vi "SubPanel_DataCollection_Rev11_v3.vi"(0 "DCPowerInformationClusterArray_Input":T1(array[cluster]), 1 "VISAPowerInfoInputArray":T7(array[cluster]), 2 "Run Data SubPanel Input":T6, 3 "RF Block Parameters":T5, 4 "Oscilloscope Info Array":T4(array[cluster]) {"vertical coupling" items=["AC", "DC", "Ground"]}, 6 "New Run?":bool, 7 "error in":errorcluster) -> (20 "DCPowerInformationClusterArray_Output":T1(array[cluster]), 21 "VISAPowerInfoInputOutput":T7(array[cluster]), 22 "Run Data SubPanel Output":T6, 23 "RF Block Parameters Output":T5, 24 "Oscilloscope Info Array Output":T4(array[cluster]) {"vertical coupling" items=["AC", "DC", "Ground"]}, 25 "Reinitialize?":bool, 26 "Data Was Collected?":bool, 27 "error out":errorcluster)   [LabVIEW 2019]
uses:
  Controls/QueueDataControl.ctl
  Controls/DataBlockControl.ctl
  Controls/QueueDataControl_V2.ctl
  Controls/RFBlockControl.ctl
  <instrlib>/niScope/Controls/niScope vertical coupling.ctl
panel:
  out "DCPowerInformationClusterArray_Input 2":T1(array[cluster])
  out "Forced Exit":bool
  out "output cluster":T2
  out "Full Run Information":string
  out "Ready For Next Run?":bool
  in  "Next Run":bool
  out "Latchup Output Data":dbl[][](array[numeric])
  out "Recording Data":bool
  out "Current 2":waveform(dbl)[](graph)
  out "Voltage 2":waveform(dbl)[](graph)
  out "Current":waveform(dbl)[](graph)
  out "Voltage":waveform(dbl)[](graph)
  in  "End Collecting":bool
  in  "Record Data Toggle":bool
  out "error of collection":errorcluster
  in  "force exit SubVI":bool
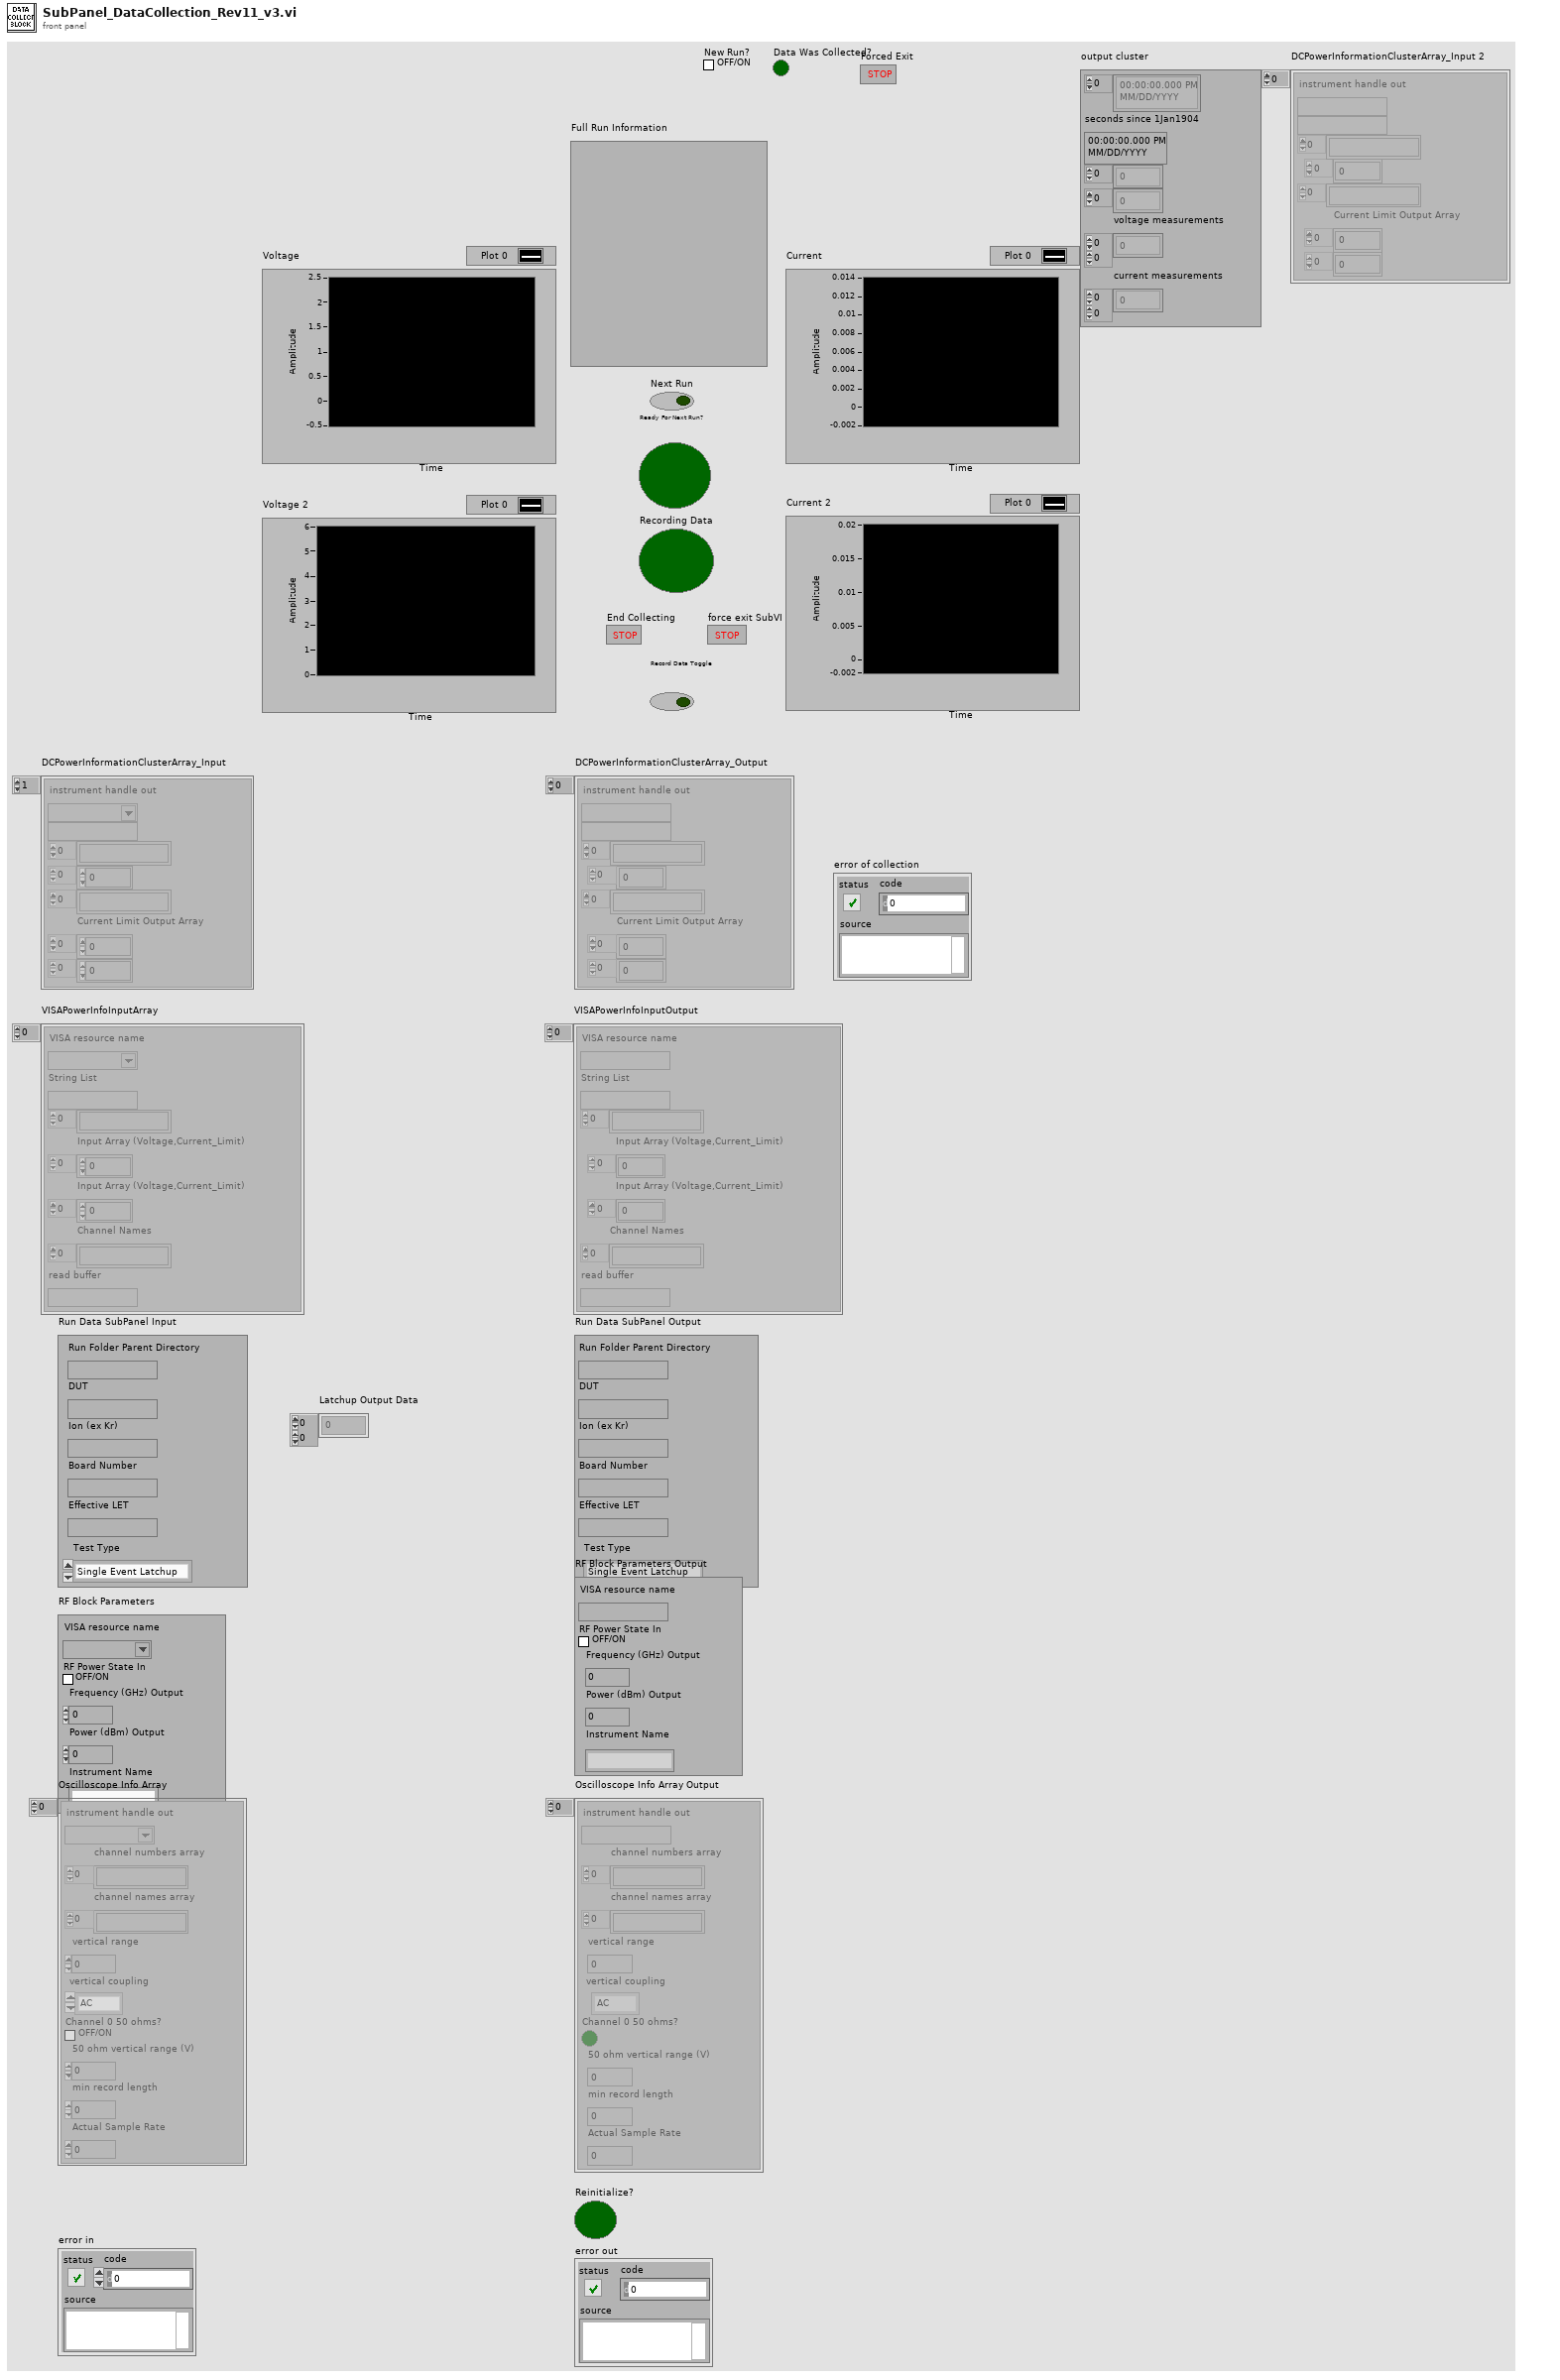
[diagram p1: front panel]
types:
  T1 = cluster{"instrument handle out":refnum<k15>, string, string[], dbl[], string[], "Current Limit Output Array":dbl[], dbl[]}[]
  T2 = cluster{timestamp[], "seconds since 1Jan1904":timestamp, dbl[], i32[], "voltage measurements":dbl[][], "current measurements":dbl[][]}
  T3 = typedef "niScope vertical coupling.ctl" = i32
  T4 = cluster{"instrument handle out":refnum<k15>, "channel numbers array":string[], "channel names array":string[], "vertical range":dbl, "vertical coupling":T3, "Channel 0 50 ohms?":bool, "50 ohm vertical range (V)":dbl, "min record length":i32, "Actual Sample Rate":dbl}[]
  T5 = typedef "RFBlockControl.ctl" = cluster{"VISA resource name":refnum<visa-resource-name>, "RF Power State In":bool, "Frequency (GHz) Output":dbl, "Power (dBm) Output":dbl, "Instrument Name":string}
  T6 = typedef "DataBlockControl.ctl" = cluster{"Run Folder Parent Directory":path, "DUT":string, "Ion (ex Kr)":string, "Board Number":string, "Effective LET":string, "Test Type":enum16{"Single Event Latchup", "Single Event Transient", "Single Event Upset"}}
  T7 = cluster{"VISA resource name":refnum<visa-resource-name>, "String List":string, string[], "Input Array (Voltage,Current_Limit)":dbl[], "Input Array (Voltage,Current_Limit)":dbl[], "Channel Names":string[], "read buffer":string}[]
  T8 = typedef "QueueDataControl_V2.ctl" = cluster{"Time Stamp Array":timestamp[], "Initial Time":timestamp, "dt measurement array":dbl[], "samples per capture":i32[], "voltage measurements":dbl[][], "current measurements":dbl[][]}
  T9 = cluster{"IVI Refnum out":refnum<k15>, string, "voltage level channel 23":dbl, "Channel Name 23":string, "Current Limit":dbl, "Measure Record dt":dbl, string}[]
  T10 = typedef "QueueDataControl.ctl" = cluster{"Rolling Timer":timestamp, "Initial Time":timestamp, "dt between samples":dbl[], "number of samples per fetch":i32[], "voltage measurements":dbl[][], "current measurements":dbl[][]}
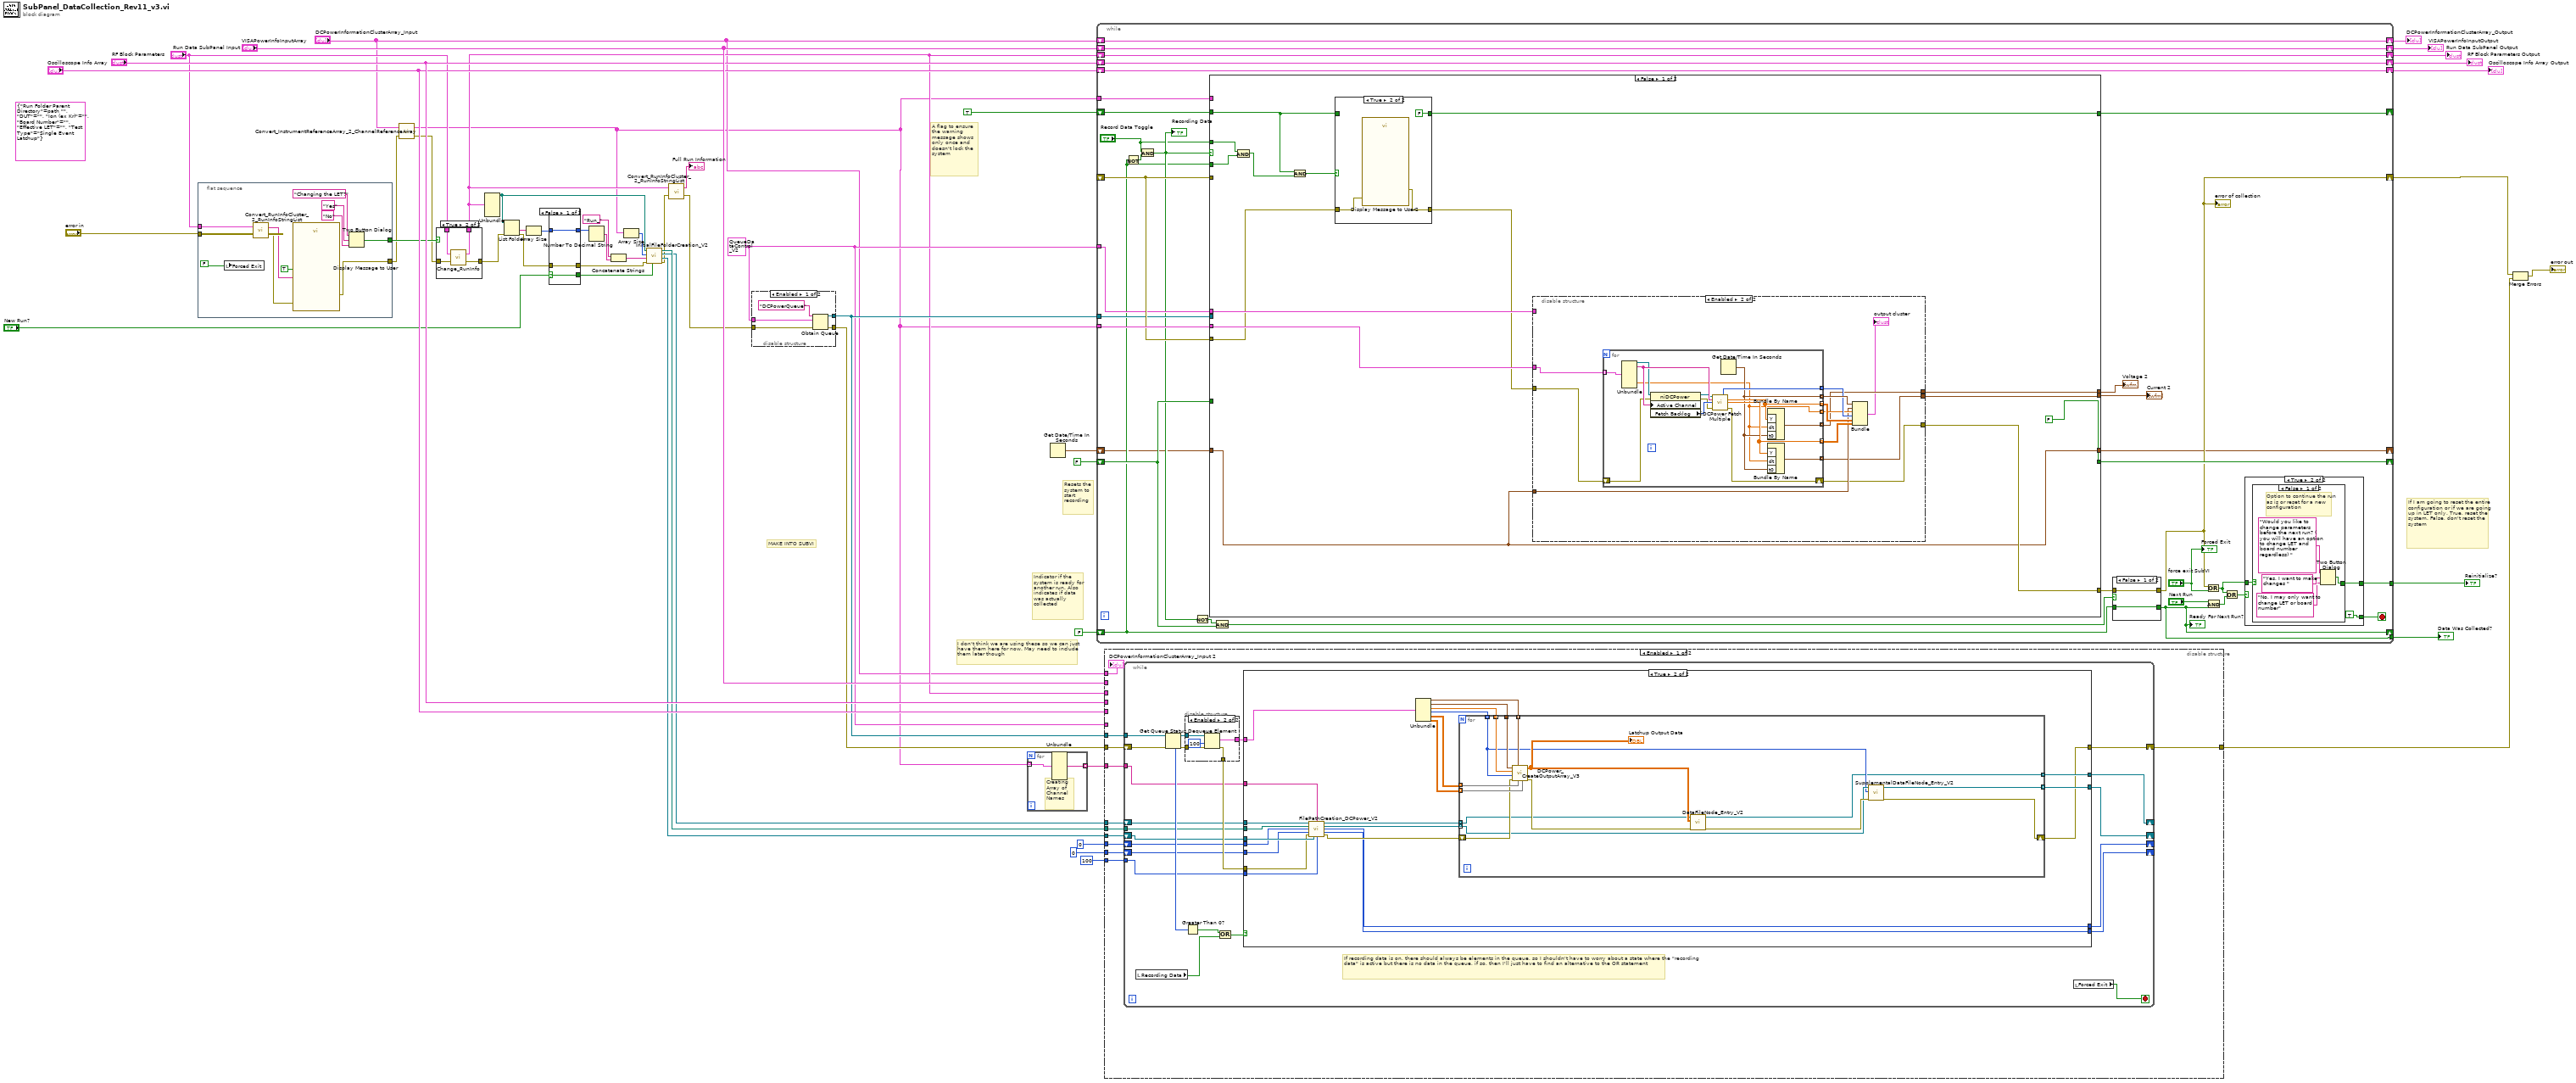
[diagram p0: block diagram]
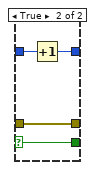
[diagram p2: hidden frame]
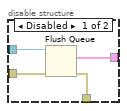
[diagram p5: hidden frame]
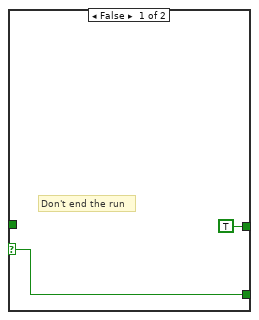
[diagram p8: hidden frame]
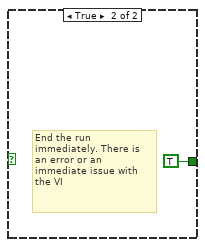
[diagram p9: hidden frame]
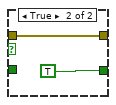
[diagram p10: hidden frame]
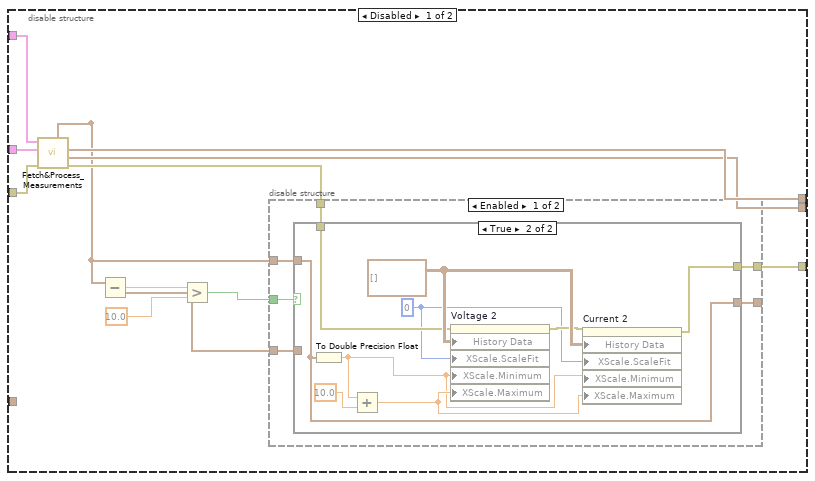
[diagram p11: hidden frame]
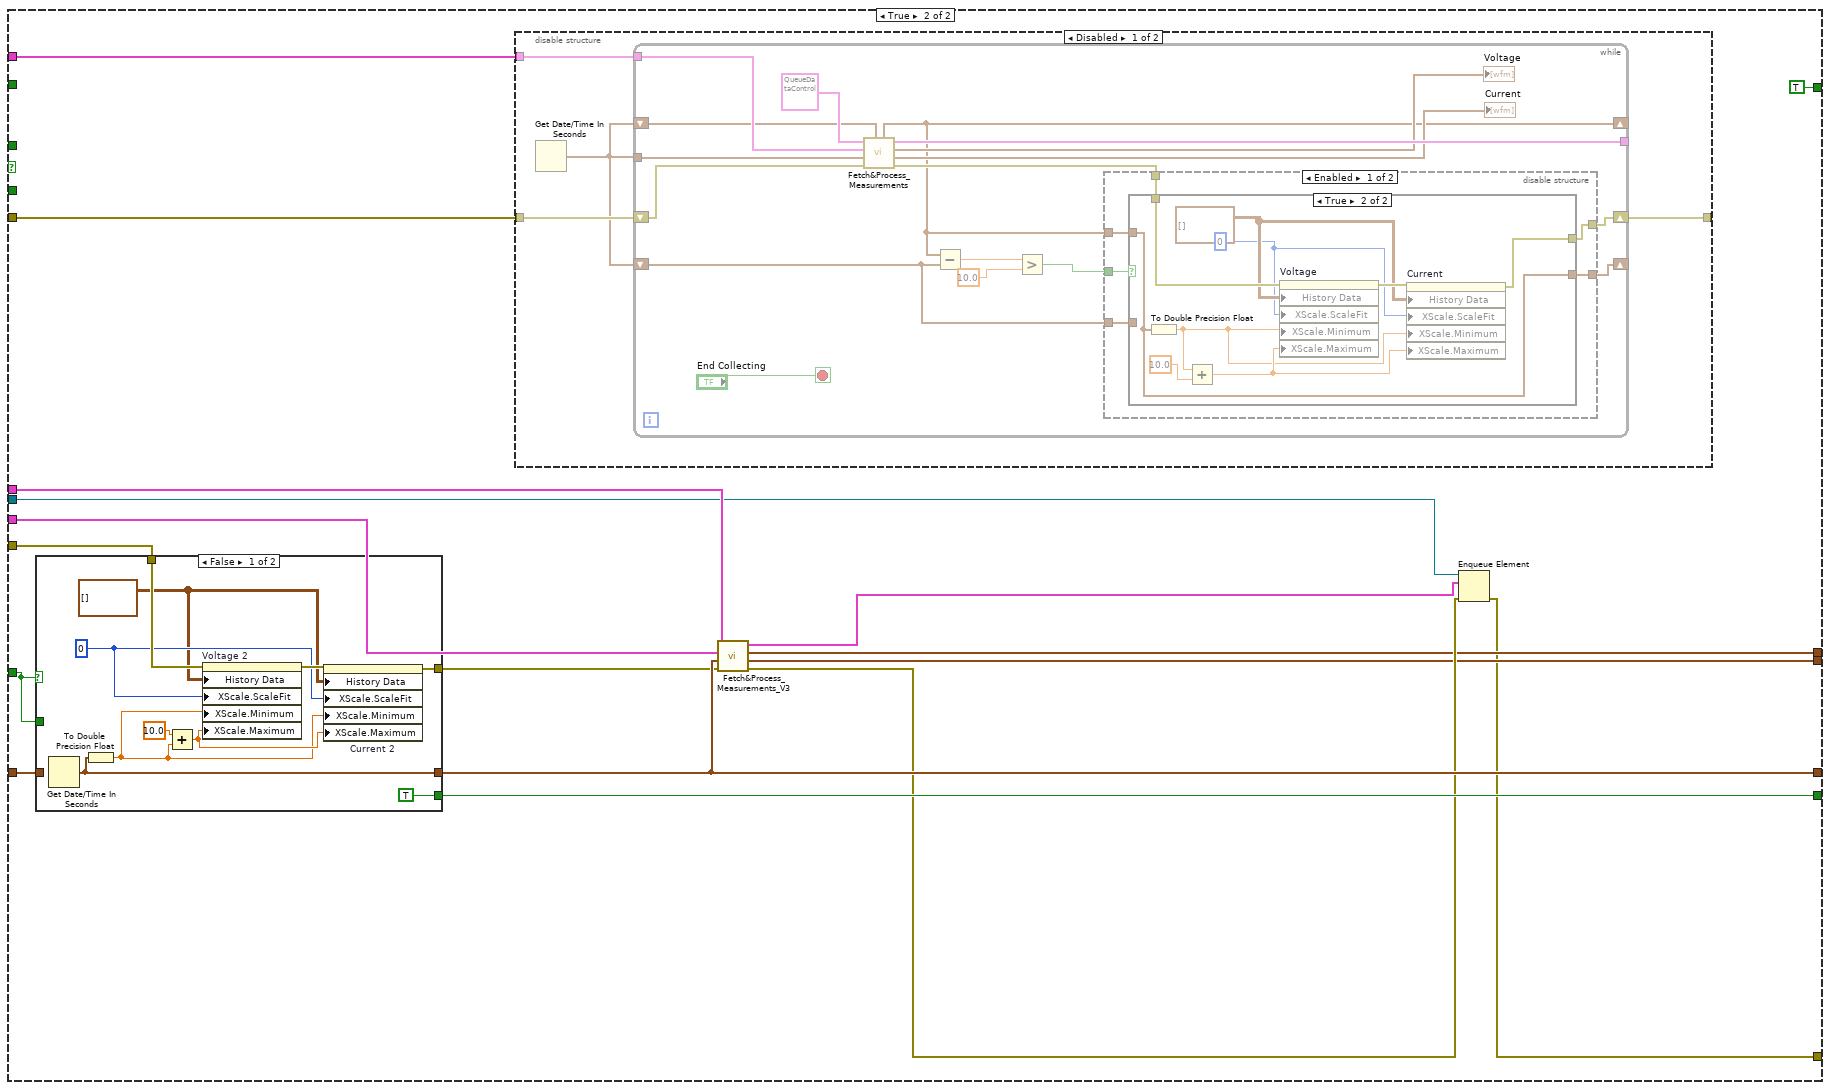
[diagram p15: hidden frame]
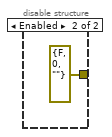
[diagram p19: hidden frame]
diagram:
  w32 = T8 {"Time Stamp Array"=[], "Initial Time"=timestamp(0 s since 1904-01-01), "dt measurement array"=[], "samples per capture"=[], "voltage measurements"=[], "current measurements"=[]} ("DCPowerDataQueueControl_V2")
  (unwired) T6 {"Run Folder Parent Directory"=path "", "DUT"="", "Ion (ex Kr)"="", "Board Number"="", "Effective LET"="", "Test Type"=enum."Single Event Latchup"} ("Run Data Configuration")
  # "I don't think we are using these so we can just have them here for now. May need to include them later though"
  # "Indicator if the system is ready for another run. Also indicates if data was actually collected"
  # "Resets the system to start recording"
  # "A flag to ensure the warning message shows only once and doesn't lock the system"
  # "If I am going to reset the entire configuration or if we are going up in LET only. True, reset the system. False, don't reset the system"
  # "MAKE INTO SUBVI"
  n1 = flat-sequence {
    tunnel: [w58] -> w26
    tunnel: "error in" -> [w57]
    tunnel: [w62] -> w36
    tunnel: "Run Data SubPanel Input" -> [w55]
    frame #0 {
      n2 = local write "Forced Exit"(FALSE ("Forced Exit")) -> ()
      n3 = call "Convert_RunInfoCluster_2_RunInfoStringList.vi"("error in"=w57, "Run Data SubPanel Input"=w55) -> ("error output"=w56:errorcluster, "Run Data Output"=w54:string)
      n4 = call "Display Message to User"("error in (no error)"=w56, "Enable"=TRUE, "Message"=w54) -> ("error out"=w58:errorcluster)  [unwired: 7 in, 1 out]
      n5 = Two Button Dialog(message="Changing the LET?", 1:"No" ("F button name (\"Cancel\")"), 2:"Yes" ("T button name (\"OK\")")) -> (T button?=w62:bool)
    }
  }
  n6 = call "Convert_InstrumentReferenceArray_2_ChannelReferenceArray.vi"("error in (no error)"=w26, "DCPowerInformationClusterArray_Input"="DCPowerInformationClusterArray_Input") -> ("error out"=w24:errorcluster, "DCPowerInformation_byChannel"=w7:T9)
  n7 = case shown="True" w36 {
    tunnel: "Run Data SubPanel Input" -> [w64 w68]
    tunnel: [w64 w67] -> w31
    tunnel: [w63 w66] -> w28
    tunnel: w24 -> [w63 w65]
    frame False {
    }
    frame True {
      n8 = call "Change_RunInfo.vi"("error in (no error)"=w65, "Run Data SubPanel in"=w68) -> ("error out"=w66:errorcluster, "Run Data SubPanel out"=w67:T6)
    }
  }
  n9 = Unbundle(w31) -> ("Run Folder Parent Directory"=w29:path)  [unwired: 5 out]
  n10 = List Folder(path=w29, error in=w28) -> (folder names=w30:string[], error out=w8:errorcluster)  [unwired: 2 in, 2 out]
  n11 = Array Size(array=w30) -> (size(s)=w11:i32)
  n12 = case shown="False" "New Run?" {
    selector: "New Run?" -> [w70 w73]
    tunnel: [w71 w75] -> w12
    tunnel: w11 -> [w71 w74]
    tunnel: [w70 w73] -> w10
    tunnel: [w69 w72] -> w9
    tunnel: w8 -> [w69 w72]
    frame False {
    }
    frame True {
      n13 = Increment(x=w74) -> (x+1=w75:i32)
    }
  }
  n14 = Number To Decimal String(number=w12) -> (decimal integer string=w16:string)  [unwired: 1 in]
  n15 = Concatenate Strings("Run_", w16) -> (w27:string)
  n16 = Array Size(array=w7) -> (size(s)=w6:i32)
  n17 = call "InitialFileFolderCreation_V2.vi"("New Run?"=w10, "error in (no error)"=w9, "Run Number"=w27, "DCPowerArrayClusterSize"=w6, "base path"=w29) -> ("error out"=w5:errorcluster, "SupplementalDataFileReferenceObjectArray"=w20:refnum<file>[], "DataFileReferenceObjectArray"=w21:refnum<file>[], "created path"=w22:path)  [unwired: 3 in]
  n18 = call "Convert_RunInfoCluster_2_RunInfoStringList.vi"("error in"=w5, "Run Data SubPanel Input"=w31) -> ("error output"=w4:errorcluster, "Run Data Output"=→"Full Run Information":string)
  n19 = disable-structure shown="Enabled" {
    disable-tunnel: w4 -> [w79 w81]
    disable-tunnel: [w78 w81] -> w41
    disable-tunnel: w32 -> [w77 _]
    disable-tunnel: [w76 _] -> w42
    frame Enabled {
      n20 = Obtain Queue(name (unnamed)="DCPowerQueue", element data type=w77, error in (no error)=w79) -> (queue out=w76:refnum<queue>, error out=w78:errorcluster)  [unwired: 2 in, 1 out]
    }
    frame Disabled {
    }
  }
  n21 = for {
    tunnel: w7 -> [w83] mode=indexing
    tunnel: [w82] -> w23 mode=indexing
    # "Creating Array of Channel Names"
    n22 = Unbundle(w83) -> ("Channel Name 23"=w82:string)  [unwired: 6 out]
  }
  n23 = Get Date/Time In Seconds() -> (seconds since 1Jan1904=w33:timestamp)
  n24 = while {
    shift-right: [w113] -> w51
    shift-left: "DCPowerInformationClusterArray_Input" -> [w113]
    shift-right: [w117] -> w50
    shift-left: "VISAPowerInfoInputArray" -> [w117]
    shift-right: [w116] -> w49
    shift-left: w31 -> [w116]
    shift-right: [w115] -> w48
    shift-left: "RF Block Parameters" -> [w115]
    shift-right: [w114] -> w47
    shift-left: "Oscilloscope Info Array" -> [w114]
    shift-right: [w96] -> w2
    shift-left: _ -> [w110]
    tunnel: w7 -> [w112]
    tunnel: w7 -> [w111]
    shift-right: [w107] -> _
    shift-left: FALSE -> [w103]
    tunnel: w32 -> [w106]
    tunnel: w42 -> [w105]
    shift-right: [w84] -> _
    shift-left: FALSE -> [w89]
    tunnel: [w93] -> w40
    shift-right: [w87] -> _
    shift-left: TRUE ("x .and. y?") -> [w88]
    shift-right: [w85] -> _
    shift-left: w33 -> [w86]
    tunnel: [w84] -> w14
    stop <- w94 stop-if-true
    n25 = Not(x=w89) -> (.not. x?=w91:bool)
    n26 = And(x="Record Data Toggle", y=w91) -> (x .and. y?=w92:bool)
    "Recording Data" <- w92
    n27 = Not(x=w92) -> (.not. x?=w104:bool)
    n28 = case shown="False" w92 {
      tunnel: w110 -> [_ w228]
      tunnel: w112 -> [_ w227]
      tunnel: w111 -> [w146 w225]
      tunnel: w110 -> [w140 w222]
      tunnel: [w143 w213] -> w109
      tunnel: [w144 w214] -> w108
      tunnel: w106 -> [w145 w218]
      tunnel: w103 -> [_ w219]
      tunnel: [FALSE w220] -> w107
      tunnel: w105 -> [_ w217]
      tunnel: [w141 w212] -> w101
      tunnel: "Record Data Toggle" -> [w137 _]
      tunnel: w89 -> [w138 _]
      tunnel: w88 -> [w133 _]
      tunnel: [w134 TRUE] -> w87
      tunnel: w86 -> [w132 w224]
      tunnel: [w132 w223] -> w85
      frame False {
        n29 = And(x=w137, y=w138) -> (x .and. y?=w136:bool)
        n30 = And(x=w133, y=w136) -> (x .and. y?=w135:bool)
        n31 = case shown="True" w135 {
          tunnel: [w208 w210] -> w139
          tunnel: w140 -> [w208 w211]
          tunnel: [w207 FALSE] -> w134
          tunnel: w133 -> [w207 _]
          frame False {
          }
          frame True {
            n32 = call "Display Message to User2"("error in (no error)"=w211) -> ("error out"=w210:errorcluster)  [unwired: 9 in, 1 out]
          }
        }
        n33 = disable-structure shown="Enabled" {
          disable-tunnel: w146 -> [w156 w186]
          disable-tunnel: w145 -> [w155 _]
          disable-tunnel: [w151 w184] -> w144
          disable-tunnel: [w150 w183] -> w143
          disable-tunnel: [w148 w182] -> w141
          disable-tunnel: w139 -> [w147 w181]
          disable-tunnel: w132 -> [_ w185]
          frame Disabled {
            n34 = call "Fetch&Process_Measurements.vi"("error in (no error)"=w147, "DCPowerInformation_byChannel"=w156, "Queue Data Parameters in"=w155) -> ("error out"=w157:errorcluster, "Current Measurement"=w150:waveform(dbl)[], "Voltage Measurement"=w151:waveform(dbl)[], "Rolling Timer Output"=w149:timestamp, "Rolling Timer Input"=w154:timestamp)  [unwired: 3 in, 1 out]
            n35 = Subtract(x=w149, y=w152) -> (x-y=w159:dbl)
            n36 = Greater?(x=w159, y=10.0) -> (0:w158:bool)
            n37 = disable-structure shown="Enabled" {
              disable-tunnel: w158 -> [w166 _]
              disable-tunnel: w157 -> [w165 w179]
              disable-tunnel: [w164 w179] -> w148
              disable-tunnel: [w163 w178] -> w153
              disable-tunnel: w149 -> [w162 w178]
              disable-tunnel: [w161 _] -> w152
              frame Enabled {
                n38 = case shown="True" w166 {
                  tunnel: w165 -> [w168 w174]
                  tunnel: [w168 w172] -> w164
                  tunnel: [w167 w176] -> w163
                  tunnel: w162 -> [_ w176]
                  tunnel: w161 -> [w167 _]
                  frame False {
                  }
                  frame True {
                    w171 = u8 0 ("X Scale.Scale Fit")
                    w175 = waveform(dbl)[][] [] ("History Data")
                    n39 = To Double Precision Float(number=w176) -> (double precision float=w169:dbl)
                    n40 = Add(x=w169, y=10.0) -> (x+y=w170:dbl)
                    n41 = property on="Voltage 2" class="WFChart (strict)"(error in=w174, "History Data"=w175, "XScale.ScaleFit"=w171, "XScale.Minimum"=w169, "XScale.Maximum"=w170) -> (error out=w173:errorcluster)  [unwired: 1 in, 1 out]
                    n42 = property on="Current 2" class="WFChart (strict)"(error in=w173, "History Data"=w175, "XScale.ScaleFit"=w171, "XScale.Minimum"=w169, "XScale.Maximum"=w170) -> (error out=w172:errorcluster)  [unwired: 1 in, 1 out]
                  }
                }
              }
              frame Disabled {
              }
            }
          }
          frame Enabled {
            n43 = for {
              tunnel: w186 -> [w206] mode=indexing
              tunnel: [w199] -> w184 mode=indexing
              tunnel: [w198] -> w183 mode=indexing
              tunnel: [w197] -> w188 mode=indexing
              tunnel: [w196] -> w190 mode=indexing
              tunnel: [w195] -> w189 mode=indexing
              tunnel: [w194] -> w191 mode=indexing
              tunnel: [w193] -> w187 mode=indexing
              shift-right: [w192] -> w182
              shift-left: w181 -> [w203]
              n44 = Unbundle(w206) -> ("IVI Refnum out"=w202:refnum<k15>, w205:string, "Measure Record dt"=w193:dbl)  [unwired: 4 out]
              n45 = property class="niDCPower"(reference=w202, error in=w203, "Active Channel"=w205) -> (reference out=w201:refnum<k15>, error out=w200:errorcluster, "Fetch Backlog"=w204:i32)
              n46 = call <instrlib>:"niDCPower Fetch Multiple.vi"("instrument handle"=w201, "channel name"=w205, "count (1)"=w204, "error in (no error)"=w200) -> ("actual count"=w197:i32, "voltage measurements"=w195:dbl[], "current measurements"=w196:dbl[], "error out"=w192:errorcluster)  [unwired: 6 in, 2 out]
              n47 = Get Date/Time In Seconds() -> (seconds since 1Jan1904=w194:timestamp)
              n48 = Bundle By Name("Y"=w195, "dt"=w193, "t0"=w194) -> (w199:waveform(dbl))  [unwired: 1 out]
              n49 = Bundle By Name("Y"=w196, "dt"=w193, "t0"=w194) -> (w198:waveform(dbl))  [unwired: 1 out]
            }
            n50 = Bundle(w191, "seconds since 1Jan1904"=w185, w187, w188, "voltage measurements"=w189, "current measurements"=w190) -> (→"output cluster":T2)  [unwired: 1 in]
          }
        }
      }
      frame True {
        n51 = case shown="False" w219 {
          tunnel: [w233 w241] -> w223
          tunnel: w224 -> [_ w241]
          tunnel: w222 -> [w238 w240]
          tunnel: [w236 w240] -> w221
          tunnel: [TRUE w239] -> w220
          tunnel: w219 -> [_ w239]
          frame False {
            w229 = waveform(dbl)[][] [] ("History Data")
            w234 = u8 0 ("X Scale.Scale Fit")
            n52 = Get Date/Time In Seconds() -> (seconds since 1Jan1904=w233:timestamp)
            n53 = To Double Precision Float(number=w233) -> (double precision float=w230:dbl)
            n54 = Add(x=10.0 ("y"), y=w230) -> (x+y=w232:dbl)
            n55 = property on="Voltage 2" class="WFChart (strict)"(error in=w238, "History Data"=w229, "XScale.ScaleFit"=w234, "XScale.Minimum"=w230, "XScale.Maximum"=w232) -> (error out=w237:errorcluster)  [unwired: 1 in, 1 out]
            n56 = property on="Current 2" class="WFChart (strict)"(error in=w237, "History Data"=w229, "XScale.ScaleFit"=w234, "XScale.Minimum"=w230, "XScale.Maximum"=w232) -> (error out=w236:errorcluster)  [unwired: 1 in, 1 out]
          }
          frame True {
          }
        }
        n57 = disable-structure shown="Disabled" {
          disable-tunnel: w228 -> [w245 _]
          disable-tunnel: w227 -> [w244 _]
          disable-tunnel: [w243 errorcluster {"status"=FALSE, "code"=0, "source"=""} ("error out")] -> _
          frame Disabled {
            n58 = Get Date/Time In Seconds() -> (seconds since 1Jan1904=w242:timestamp)
            n59 = while {
              shift-right: [w249] -> w243
              shift-left: w245 -> [w260]
              tunnel: w244 -> [w261]
              tunnel: w242 -> [w257]
              shift-right: [w247] -> _
              shift-left: w242 -> [w258]
              tunnel: [w256] -> _
              shift-right: [w248] -> _
              shift-left: w242 -> [w246]
              stop <- "End Collecting" stop-if-true
              n60 = call "Fetch&Process_Measurements.vi"("Rolling Timer Input"=w258, "error in (no error)"=w260, "Initial Time"=w257, "DCPowerInformation_byChannel"=w261, "Queue Data Parameters in"=T10 {"Rolling Timer"=timestamp(0 s since 1904-01-01), "Initial Time"=timestamp(0 s since 1904-01-01), "dt between samples"=[], "number of samples per fetch"=[], "voltage measurements"=[], "current measurements"=[]} ("Queue Data Parameters")) -> ("error out"=w250:errorcluster, "Current Measurement"=→"Current":waveform(dbl)[], "Voltage Measurement"=→"Voltage":waveform(dbl)[], "Queue Data Parameters out"=w256:T10, "Rolling Timer Output"=w247:timestamp)  [unwired: 2 in]
              n61 = Subtract(x=w247, y=w246) -> (x-y=w252:dbl)
              n62 = Greater?(x=w252, y=10.0) -> (0:w251:bool)
              n63 = disable-structure shown="Enabled" {
                disable-tunnel: w251 -> [w268 _]
                disable-tunnel: w250 -> [w267 w281]
                disable-tunnel: [w266 w281] -> w249
                disable-tunnel: [w265 w280] -> w248
                disable-tunnel: w247 -> [w264 w280]
                disable-tunnel: w246 -> [w263 _]
                frame Enabled {
                  n64 = case shown="True" w268 {
                    tunnel: w267 -> [w270 w279]
                    tunnel: [w270 w277] -> w266
                    tunnel: [w269 w271] -> w265
                    tunnel: w264 -> [_ w271]
                    tunnel: w263 -> [w269 _]
                    frame False {
                    }
                    frame True {
                      w274 = u8 0 ("X Scale.Scale Fit")
                      w275 = waveform(dbl)[][] [] ("History Data")
                      n65 = To Double Precision Float(number=w271) -> (double precision float=w272:dbl)
                      n66 = Add(x=w272, y=10.0) -> (x+y=w273:dbl)
                      n67 = property on="Voltage" class="WFChart (strict)"(error in=w279, "History Data"=w275, "XScale.ScaleFit"=w274, "XScale.Minimum"=w272, "XScale.Maximum"=w273) -> (error out=w278:errorcluster)  [unwired: 1 in, 1 out]
                      n68 = property on="Current" class="WFChart (strict)"(error in=w278, "History Data"=w275, "XScale.ScaleFit"=w274, "XScale.Minimum"=w272, "XScale.Maximum"=w273) -> (error out=w277:errorcluster)  [unwired: 1 in, 1 out]
                    }
                  }
                }
                frame Disabled {
                }
              }
            }
          }
          frame Enabled {
          }
        }
        n69 = call "Fetch&Process_Measurements_V3.vi"("error in (no error)"=w221, "Initial Time"=w223, "DCPowerInformation_byChannel"=w225, "DCPowerDataQueueControl_V2 in"=w218) -> ("error out"=w216:errorcluster, "Current Waveform"=w213:waveform(dbl)[], "Voltage Waveform"=w214:waveform(dbl)[], "DCPowerDataQueueControl_V2 out"=w215:T8)  [unwired: 4 in]
        n70 = Enqueue Element(queue=w217, element=w215, error in (no error)=w216) -> (error out=w212:errorcluster)  [unwired: 1 in, 2 out]
      }
    }
    "Voltage 2" <- w108
    "Current 2" <- w109
    n71 = And(x=w104, y=w103) -> (x .and. y?=w102:bool)
    n72 = case shown="False" w102 {
      tunnel: w101 -> [w128 w130]
      tunnel: [w129 TRUE] -> w84
      tunnel: w89 -> [w129 _]
      tunnel: [w128 w130] -> w96
      frame False {
      }
      frame True {
      }
    }
    "error of collection" <- w96
    "Ready For Next Run?" <- w84
    n73 = Or(x=w96, y="force exit SubVI") -> (x .or. y?=w98:bool)
    n74 = And(x="Next Run", y=w84) -> (x .and. y?=w100:bool)
    n75 = Or(x=w98, y=w100) -> (x .or. y?=w99:bool)
    n76 = case shown="True" w99 {
      selector: w99 -> [w119 _]
      tunnel: w98 -> [_ w122]
      tunnel: [w119 TRUE] -> w94
      tunnel: [TRUE ("T button?") w120] -> w93
      frame False {
        # "Don't end the run"
      }
      frame True {
        n77 = case shown="False" w122 {
          tunnel: [w123 TRUE] -> w120
          frame False {
            # "Option to continue the run as is or reset for a new configuration"
            n78 = Two Button Dialog(message="Would you like to change parameters before the next run? ( you will have an option to change LET and board number regardless) ", 1:"No, I may only want to change LET or board number" ("F button name (\"Cancel\")"), 2:"Yes, I want to make changes " ("T button name (\"OK\")")) -> (T button?=w123:bool)
          }
          frame True {
            # "End the run immediately. There is an error or an immediate issue with the VI"
          }
        }
      }
    }
    "Forced Exit" <- "force exit SubVI"
  }
  "DCPowerInformationClusterArray_Output" <- w51
  "VISAPowerInfoInputOutput" <- w50
  "Run Data SubPanel Output" <- w49
  "RF Block Parameters Output" <- w48
  "Oscilloscope Info Array Output" <- w47
  "Reinitialize?" <- w40
  "Data Was Collected?" <- w14
  n79 = disable-structure shown="Enabled" {
    disable-tunnel: "DCPowerInformationClusterArray_Input" -> [w284 _]
    disable-tunnel: "VISAPowerInfoInputArray" -> [_ _]
    disable-tunnel: w31 -> [_ _]
    disable-tunnel: "RF Block Parameters" -> [_ _]
    disable-tunnel: "Oscilloscope Info Array" -> [_ _]
    disable-tunnel: w42 -> [w293 _]
    disable-tunnel: w41 -> [w292 _]
    disable-tunnel: w32 -> [_ _]
    disable-tunnel: w23 -> [w291 _]
    disable-tunnel: w22 -> [w290 _]
    disable-tunnel: w21 -> [w289 _]
    disable-tunnel: w20 -> [w288 _]
    disable-tunnel: 0 ("binary file indexor in") -> [w287 _]
    disable-tunnel: 0 ("binary file indexor in") -> [w286 _]
    disable-tunnel: 100 ("binary file indexor in") -> [w285 _]
    disable-tunnel: [w283 _] -> w3
    frame Enabled {
      n80 = while {
        tunnel: w293 -> [w308]
        shift-right: [w295] -> w283
        shift-left: w292 -> [w307]
        tunnel: w290 -> [w304]
        shift-right: [w297] -> _
        shift-left: w289 -> [w305]
        shift-right: [w296] -> _
        shift-left: w288 -> [w303]
        shift-right: [w299] -> _
        shift-left: w287 -> [w302]
        shift-right: [w298] -> _
        shift-left: w286 -> [w301]
        tunnel: w285 -> [w300]
        tunnel: w291 -> [w306]
        stop <- w294 stop-if-true
        # "If recording data is on, there should always be elements in the queue, so I shouldn't have to worry about a state where the \"recording data\" is active but there is no data in the queue, if so, then I'll just have to find an alternative to the OR statement"
        n81 = local read "Recording Data"() -> (w313:bool)
        n82 = Get Queue Status(queue=w308, error in (no error)=w307) -> (queue out=w310:refnum<queue>, error out=w311:errorcluster, # elements in queue=w316:i32)  [unwired: 1 in, 5 out]
        n83 = disable-structure shown="Enabled" {
          disable-tunnel: [w320 w322] -> w312
          disable-tunnel: w311 -> [w319 w324]
          disable-tunnel: w310 -> [w318 w325]
          disable-tunnel: [w317 w321] -> w309
          frame Disabled {
            n84 = Flush Queue(queue=w318, error in (no error)=w319) -> (remaining elements=w317:T8[], error out=w320:errorcluster)  [unwired: 1 out]
          }
          frame Enabled {
            n85 = Dequeue Element(queue=w325, timeout in ms (-1)=100, error in (no error)=w324) -> (element=w321:T8, error out=w322:errorcluster)  [unwired: 2 out]
          }
        }
        n86 = Greater Than 0?(x=w316) -> (x > 0?=w314:bool)
        n87 = Or(x=w314, y=w313) -> (x .or. y?=w315:bool)
        n88 = case shown="True" w315 {
          tunnel: w309 -> [_ w353]
          tunnel: w312 -> [w328 w346]
          tunnel: w306 -> [_ w352]
          tunnel: w305 -> [w329 w351]
          tunnel: w304 -> [_ w350]
          tunnel: w303 -> [w330 w349]
          tunnel: w302 -> [w327 w348]
          tunnel: w301 -> [w326 w345]
          tunnel: w300 -> [_ w344]
          tunnel: [w327 w343] -> w299
          tunnel: [w326 w342] -> w298
          tunnel: [w329 w339] -> w297
          tunnel: [w330 w338] -> w296
          tunnel: [w328 w337] -> w295
          frame False {
          }
          frame True {
            n89 = call "FilePathCreation_DCPower_V2.vi"("binary file input reference array 1"=w351, "Channel Name Input array"=w352, "data output directory folder"=w350, "binary file indexor in"=w348, "Reset counter in"=w345, "error in (no error)"=w346, "binary file input reference array 2"=w349, "reset threshold"=w344) -> ("binary file output reference array"=w341:refnum<file>[], "binary file output reference array 2"=w340:refnum<file>[], "binary file indexor out"=w343:i32, "reset counter out"=w342:i32, "error out"=w347:errorcluster)  [unwired: 3 in]
            n90 = Unbundle(w353) -> ("Time Stamp Array"=w331:timestamp[], "Initial Time"=w332:timestamp, "dt measurement array"=w336:dbl[], "samples per capture"=w335:i32[], "voltage measurements"=w334:dbl[][], "current measurements"=w333:dbl[][])
            n91 = for {
              tunnel: w336 -> [w366] mode=indexing
              tunnel: w335 -> [w356] mode=indexing
              tunnel: w334 -> [w365] mode=indexing
              tunnel: w333 -> [w364] mode=indexing
              tunnel: w332 -> [w367]
              tunnel: w331 -> [w368] mode=indexing
              shift-right: [w358] -> w337
              shift-left: w347 -> [w363]
              tunnel: w341 -> [w360] mode=indexing
              tunnel: w340 -> [w357] mode=indexing
              tunnel: [w355] -> w339 mode=indexing
              tunnel: [w354] -> w338 mode=indexing
              n92 = call "DCPower_CreateOutputArray_V3.vi"("current measurements"=w364, "voltage measurements"=w365, "Time Stamp Array"=w368, "error in"=w363, "actual count"=w356, "Measure Record dt"=w366, "Initial Time"=w367) -> ("error out"=w362:errorcluster, "Data Output Array"=w361:dbl[][])  [unwired: 3 in]
              "Latchup Output Data" <- w361
              n93 = call "DataFileNode_Entry_V2.vi"("error in (no error)"=w362, "Data Output Array"=w361, "Byte Stream File in"=w360) -> ("error out"=w359:errorcluster, "Byte Stream File out"=w355:refnum<file>)  [unwired: 7 in]
              n94 = call "SupplementalDataFileNode_Entry_V2.vi"("error in (no error)"=w359, "actual count"=w356, "Byte Stream File in"=w357) -> ("error out"=w358:errorcluster, "Byte Stream File out"=w354:refnum<file>)  [unwired: 7 in]
            }
          }
        }
        n95 = local read "Forced Exit"() -> (w294:bool)
      }
      "DCPowerInformationClusterArray_Input 2" <- w284
    }
    frame Disabled {
    }
  }
  n96 = Merge Errors(w2, w3) -> (→"error out":errorcluster)
